vi "test.vi"() -> ()   [LabVIEW 2012]
uses:
  <vilib>/robotics/Starter Kit/2.0/9632 Host Interface/NI_Robotics_Starter Kit Host_9632_2.0.lvclass
  <vilib>/robotics/Starter Kit/Host Interface/NI_Robotics_Starter Kit Host.lvclass
panel:
  out "Wz":dbl
  out "speed":dbl
  out "sign":i32
  out "b":i32
  out "a":dbl
  out "Degrees":dbl
  out "Angle":dbl
  in  "x":i32
  in  "y":i32
  out "error out":errorcluster
  in  "stop":bool
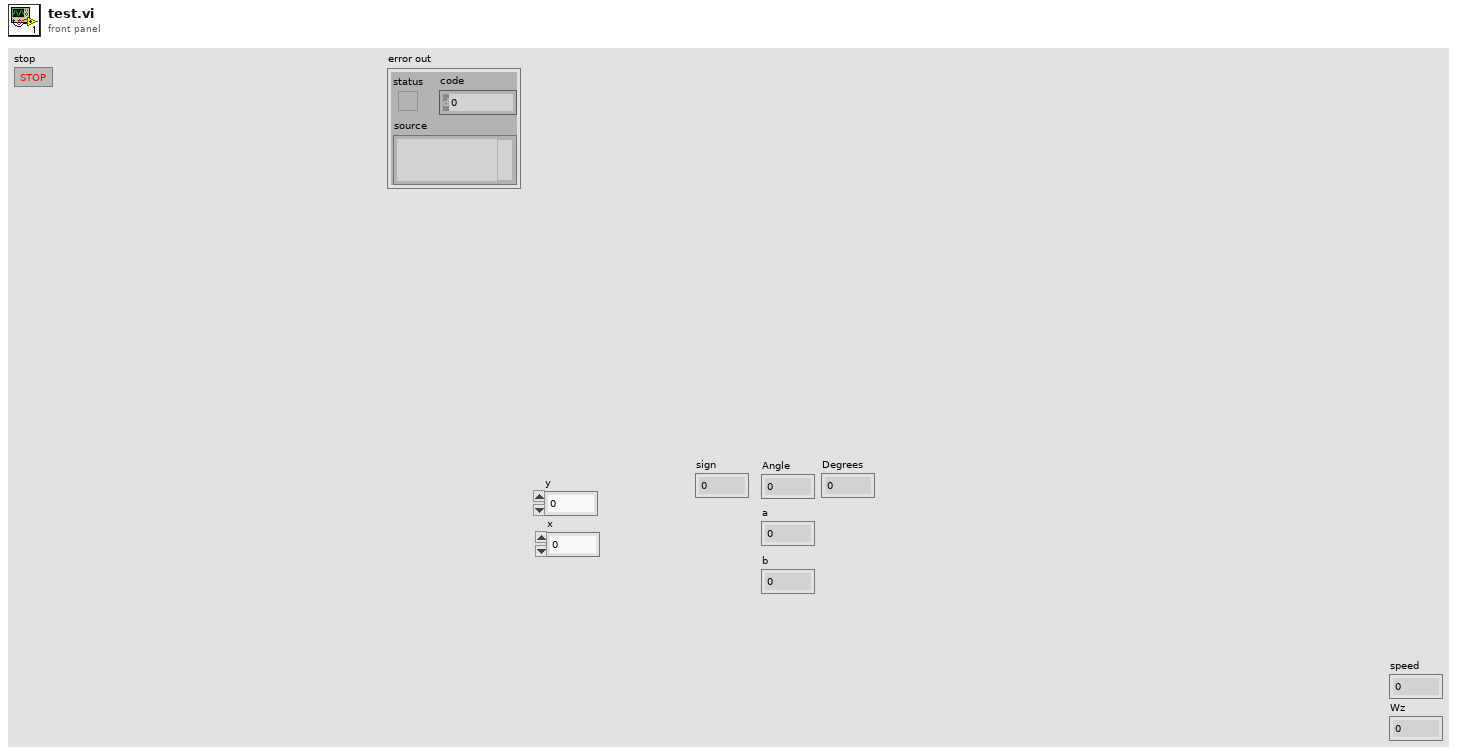
[diagram p1: front panel]
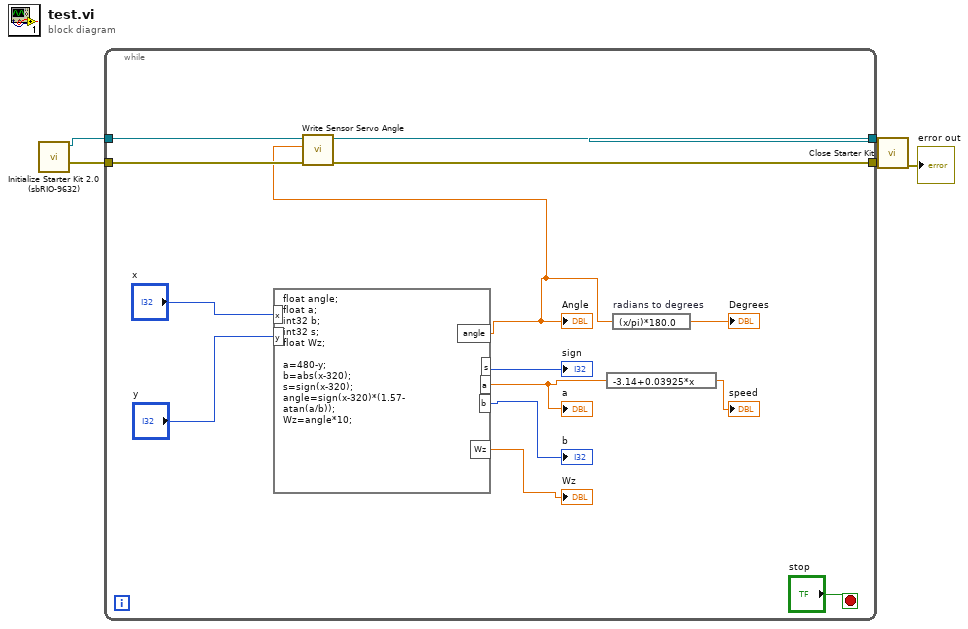
[diagram p0: block diagram]
diagram:
  n1 = call <vilib>:"Initialize Starter Kit 2.0 (sbRIO-9632).vi"() -> ("error out"=w3:errorcluster, "FPGA starter kit host 2.0 out"=w5:refnum<class "NI_Robotics_Starter Kit Host_9632_2.0.lvclass">)  [unwired: 10 in]
  n2 = while {
    tunnel: w5 -> [w18]
    tunnel: [w17] -> w4
    tunnel: w3 -> [w16]
    tunnel: [w15] -> w2
    stop <- "stop" stop-if-true
    n3 = formula code="float angle;\nfloat a;\nint32 b;\nint32 s;\nfloat Wz;\n\na=480-y;\nb=abs(x-320);\ns=sign(x-320);\nangle=sign(x-320)*(1.57-\natan(a/b));\nWz=angle*10;"("x"="x", "y"="y") -> ("angle"=w6:dbl, "a"=w12:dbl, "b"=→"b":i32, "s"=→"sign":i32, "Wz"=→"Wz":dbl)
    "Angle" <- w6
    "a" <- w12
    n4 = call <vilib>:"Write Sensor Servo Angle.vi"("error in (no error)"=w16, "ccw servo angle (rad)"=w6, "starter kit host in"=w18) -> ("error out"=w15:errorcluster, "starter kit host out"=w17:refnum<class "NI_Robotics_Starter Kit Host_9632_2.0.lvclass">)  [unwired: 7 in]
    n5 = expression code="-3.14+0.03925*x"(w12) -> (→"speed":dbl)
    n6 = expression code="(x/pi)*180.0" "radians to degrees"(w6) -> (→"Degrees":dbl)
  }
  n7 = call-dynamic "Close Starter Kit.vi"("error in (no error)"=w2, "starter kit host in"=w4) -> ("error out"=→"error out":errorcluster)  [unwired: 9 in]
